vi "ADCPinsertvalue.vi"(8 "错误输入（无错误）":errorcluster, 11 "采集数据":T2) -> (0 "错误输出":errorcluster)   [LabVIEW 2016, in "ADCP.lvlib"]
uses:
  ADCP.lvlib
panel:
  out "数组":variant[](array[variant])
  in  "data":T1
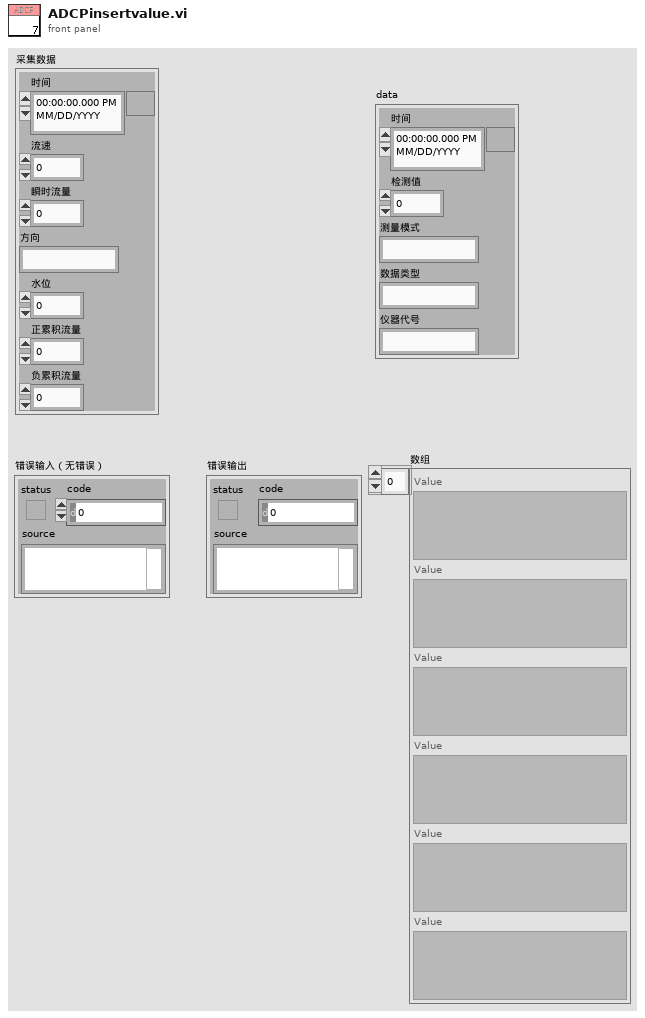
[diagram p1: front panel]
types:
  T1 = cluster{"时间":timestamp, "检测值":dbl, "测量模式":string, "数据类型":string, "仪器代号":string}
  T2 = cluster{"时间":timestamp, "流速":dbl, "瞬时流量":dbl, "方向":string, "水位":dbl, "正累积流量":dbl, "负累积流量":dbl}
  T3 = cluster{"columns外部输入":bool, "columns input":string[]}
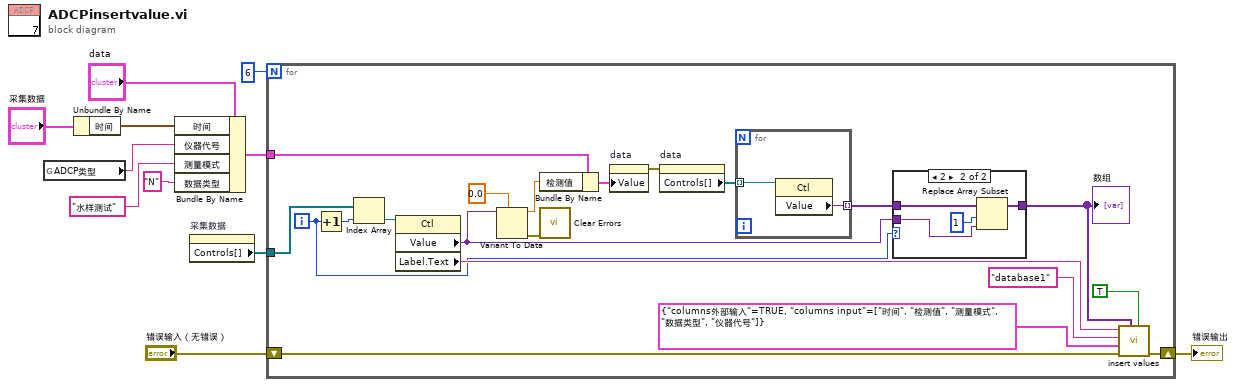
[diagram p0: block diagram]
diagram:
  n1 = global read "ADCP全局变量.vi" "ADCP类型"() -> (w1:string)
  n2 = Unbundle By Name("采集数据") -> ("时间"=w8:timestamp)
  n3 = Bundle By Name(cluster="data", "时间"=w8, "仪器代号"=w1, "测量模式"="水样测试", "数据类型"="N") -> (w7:T1)
  n4 = property on="采集数据" class="Clust (strict)"() -> ("Controls[]"=w4:refnum<vi>[])  [unwired: 2 in, 2 out]
  n5 = for {
    N: 6 -> [_]
    tunnel: w7 -> [w29]
    tunnel: w4 -> [w27]
    shift-right: [w15] -> w2
    shift-left: "错误输入（无错误）" -> [w21]
    i -> [w14]
    n6 = Increment(x=w14) -> (x+1=w31:i32)
    n7 = Index Array(array=w27, index=w31) -> (element=w30:refnum<vi>)
    n8 = property class="Ctl"(reference=w30) -> ("Value"=w19:variant, "Label.Text"=w22:string)  [unwired: 1 in, 2 out]
    n9 = Variant To Data(type=0.0, Variant=w19) -> (data=w28:dbl, error out=w16:errorcluster)  [unwired: 1 in]
    n10 = Bundle By Name(cluster=w29, "检测值"=w28) -> (w26:T1)
    n11 = call <vilib>:"Clear Errors.vi"("error in (no error)"=w16) -> ()  [unwired: 5 in, 2 out]
    n12 = property on="data" class="Clust (strict)"("Value"=w26) -> (error out=w25:errorcluster)  [unwired: 2 in, 1 out]
    n13 = property on="data" class="Clust (strict)"(error in=w25) -> ("Controls[]"=w24:refnum<vi>[])  [unwired: 1 in, 2 out]
    n14 = for {
      tunnel: w24 -> [w38] mode=indexing
      tunnel: [w37] -> w18 mode=indexing
      n15 = property class="Ctl"(reference=w38) -> ("Value"=w37:variant)  [unwired: 1 in, 2 out]
    }
    n16 = case shown="2" w14 {
      tunnel: w19 -> [_ w33]
      tunnel: w18 -> [w32 w36]
      tunnel: [w32 w34] -> w17
      frame 0, Default {
      }
      frame 2 {
        n17 = Replace Array Subset(array=w36, new element=w33, index=1 ("索引")) -> (w34:variant[])
      }
    }
    "数组" <- w17
    n18 = call "insert values.vi"("是否创建唯一键"=TRUE, "data"=w17, "错误输入（无错误）"=w21, "columns外部输入"=T3 {"columns外部输入"=TRUE, "columns input"=["时间", "检测值", "测量模式", "数据类型", "仪器代号"]}, "database"="database1", "Tabe Name"=w22) -> ("错误输出"=w15:errorcluster)  [unwired: 5 in]
  }
  "错误输出" <- w2
